vi "WriteEndOfRange.vi"(8 "ErrorIn":errorcluster caption="Error In(no Error)", 10 "MaxErrorCode":i32, 11 "ReferenceIn":refnum<class "ErrorDefinitionSQLite.lvclass"> caption="Reference In") -> (0 "ErrorOut":errorcluster caption="Error Out", 3 "ReferenceOut":refnum<class "ErrorDefinitionSQLite.lvclass"> caption="Reference Out")   [LabVIEW 2021, in "ErrorDefinitionSQLite.lvclass"]
uses:
  ErrorDefinitionSQLite.lvclass
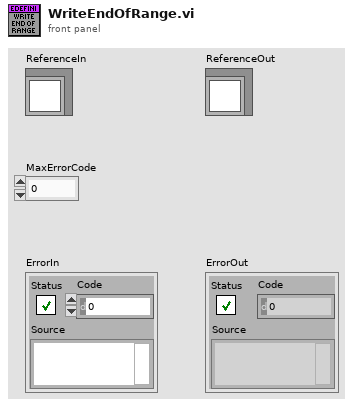
[diagram p1: front panel]
types:
  T1 = typedef "ErrorDefinitionSQLite.lvclass/ObjectAttributes.ctl" = cluster{"Path":path, "SQLiteRef":refnum<class "Connection.lvclass">, "EndOfRange":i32, "StartOfRange":i32}
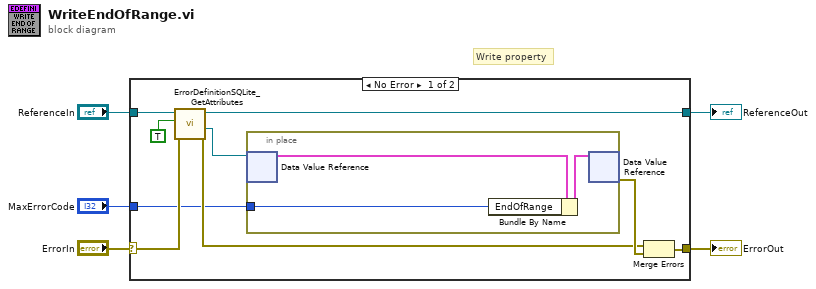
[diagram p0: block diagram]
diagram:
  # "Write property"
  n1 = case shown="No Error" "ErrorIn" {
    selector: "ErrorIn" -> [w12 w19]
    tunnel: [w13 w19] -> w4
    tunnel: [w8 w18] -> w2
    tunnel: "ReferenceIn" -> [w9 w18]
    tunnel: "MaxErrorCode" -> [w10 _]
    frame No Error {
      n2 = call "ErrorDefinitionSQLite_GetAttributes.vi"("ErrorIn"=w12, "OnlyGetDVRReference"=TRUE ("OnlyGetDvrReference(False)"), "ReferenceIn"=w9) -> ("ErrorOut"=w11:errorcluster, "DataRef"=w7:refnum<data-value>, "ReferenceOut"=w8:refnum<class "ErrorDefinitionSQLite.lvclass">)  [unwired: 5 in, 1 out]
      n3 = in-place {
        in-place-border: w10 -> [w17]
        n4 = in-place-dvr #1(w7) -> (w16:T1)  [unwired: 1 out]
        n5 = Bundle By Name(cluster=w16, "EndOfRange"=w17) -> (w15:T1)
        n6 = in-place-dvr #1(w15) -> (w14:errorcluster)  [unwired: 1 out]
      }
      n7 = Merge Errors(w11, w14) -> (w13:errorcluster)
    }
    frame Error {
    }
  }
  "ErrorOut" <- w4
  "ReferenceOut" <- w2
